vi "Oscillator Counts to Length.vi"(9 "All Temps":dbl[](array[numeric]), 10 "Oscillator freq":i32=3686400, 11 "Controller Output":string) -> (0 "Avg Range":dbl, 1 "Range STD":dbl, 3 "Distance to Cal Hole":dbl)   [LabVIEW 2014]
uses:
  Acquisition/Acquisition.lvlib
  Analysis/Analysis.lvlib
panel:
  in  "Humidity":dbl=60.0 format="%0.3f"
  out "Error (mm) at 5 m":dbl format="%#_4g"
  out "Error (mm) at 10 m":dbl format="%#_4g"
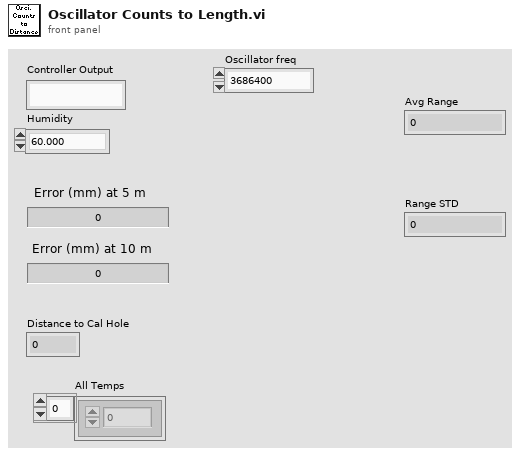
[diagram p1: front panel]
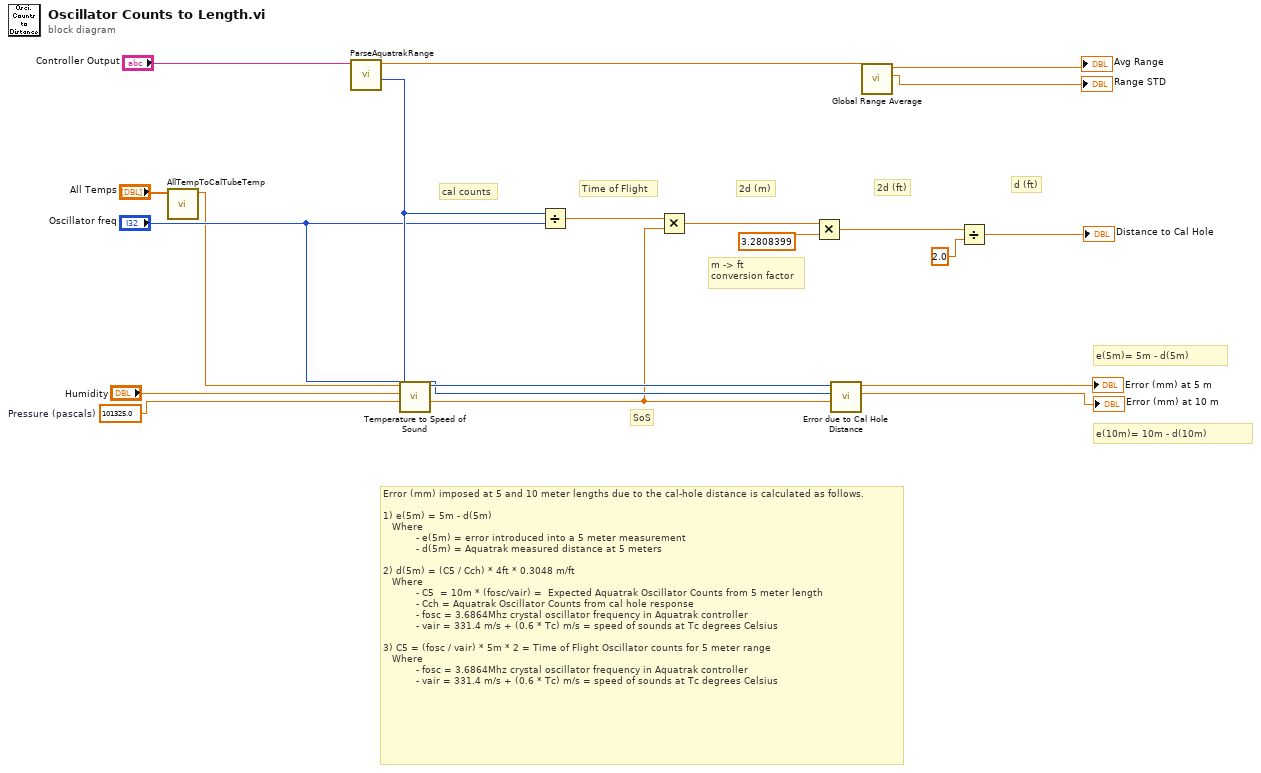
[diagram p0: block diagram]
diagram:
  w1 = 101325.0  # Pressure (pascals)
  # "d (ft)"
  # "2d (ft)"
  # "Time of Flight"
  # "2d (m)"
  # "m -> ft\nconversion factor"
  # "e(10m)= 10m - d(10m)"
  # "e(5m)= 5m - d(5m)"
  # "Error (mm) imposed at 5 and 10 meter lengths due to the cal-hole distance is calculated as follows.\n\n1) e(5m) = 5m - d(5m)\n   Where\n           - e(5m) = error introduced into a 5 meter measurement\n           - d(5m) = Aquatrak measured distance at 5 meters\n\n2) d(5m) = (C5 / Cch) * 4ft * 0.3048 m/ft\n   Where\n           - C5  = 10m * (fosc/vair) =  Expected Aquatrak Oscillator Counts from 5 meter length\n           - Cch = Aquatrak Oscillator Counts from cal hole response\n           - fosc = 3.6864Mhz crystal oscillator frequency in Aquatrak controller\n           - vair = 331.4 m/s + (0.6 * Tc) m/s = speed of sounds at Tc degrees Celsius\n\n3) C5 = (fosc / vair) * 5m * 2 = Time of Flight Oscillator counts for 5 meter range\n   Where\n           - fosc = 3.6864Mhz crystal oscillator frequency in Aquatrak controller\n           - vair = 331.4 m/s + (0.6 * Tc) m/s = speed of sounds at Tc degrees Celsius"
  # "SoS"
  # "cal counts"
  n1 = call "AllTempToCalTubeTemp.vi"("All Temps"="All Temps") -> ("Cal Tube Temps"=w4:dbl)  [unwired: 10 in]
  n2 = call "ParseAquatrakRange.vi"("Incoming String"="Controller Output") -> ("Cal Counts"=w9:i32, "Range"=w3:dbl)  [unwired: 6 in, 3 out]
  n3 = call "Temperature to Speed of Sound.vi"("Pressure (pascals)"=w1, "Humidity"="Humidity", "Temperature"=w4) -> ("Cramer Speed of Sound at Tc Humid Air (m/s)"=w6:dbl)  [unwired: 7 in, 1 out]
  n4 = Divide(x=w9, y="Oscillator freq") -> (x/y=w19:dbl)
  n5 = Multiply(x=w19, y=w6) -> (x*y=w17:dbl)
  n6 = Multiply(x=w17, y=3.2808399) -> (x*y=w16:dbl)
  n7 = call "Error due to Cal Hole Distance.vi"("Speed of Sound at Tc"=w6, "Oscillator freq"="Oscillator freq", "Cal Counts"=w9) -> ("mm Error @ 10m"=→"Error (mm) at 10 m":dbl, "mm Error @ 5m"=→"Error (mm) at 5 m":dbl)  [unwired: 7 in]
  n8 = call "Global Range Average.vi"("Range In"=w3) -> ("Std"=→"Range STD":dbl, "Average Range"=→"Avg Range":dbl)  [unwired: 9 in]
  n9 = Divide(x=w16, y=2.0) -> (x/y=→"Distance to Cal Hole":dbl)
